vi "Header Fill Check.vi"(8 "error in (no error)":errorcluster, 11 "Sample Properties:":T1) -> (0 "error out":errorcluster, 3 "Cluster":T1)   [LabVIEW 2012]
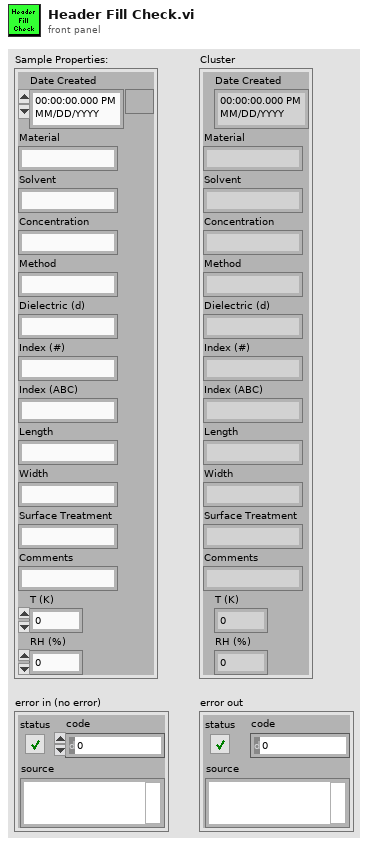
[diagram p1: front panel]
types:
  T1 = cluster{"Date Created":timestamp, "Material":string, "Solvent":string, "Concentration":string, "Method":string, "Dielectric (d)":string, "Index (#)":string, "Index (ABC)":string, "Length":string, "Width":string, "Surface Treatment":string, "Comments":string, "T (K)":dbl, "RH (%)":dbl}
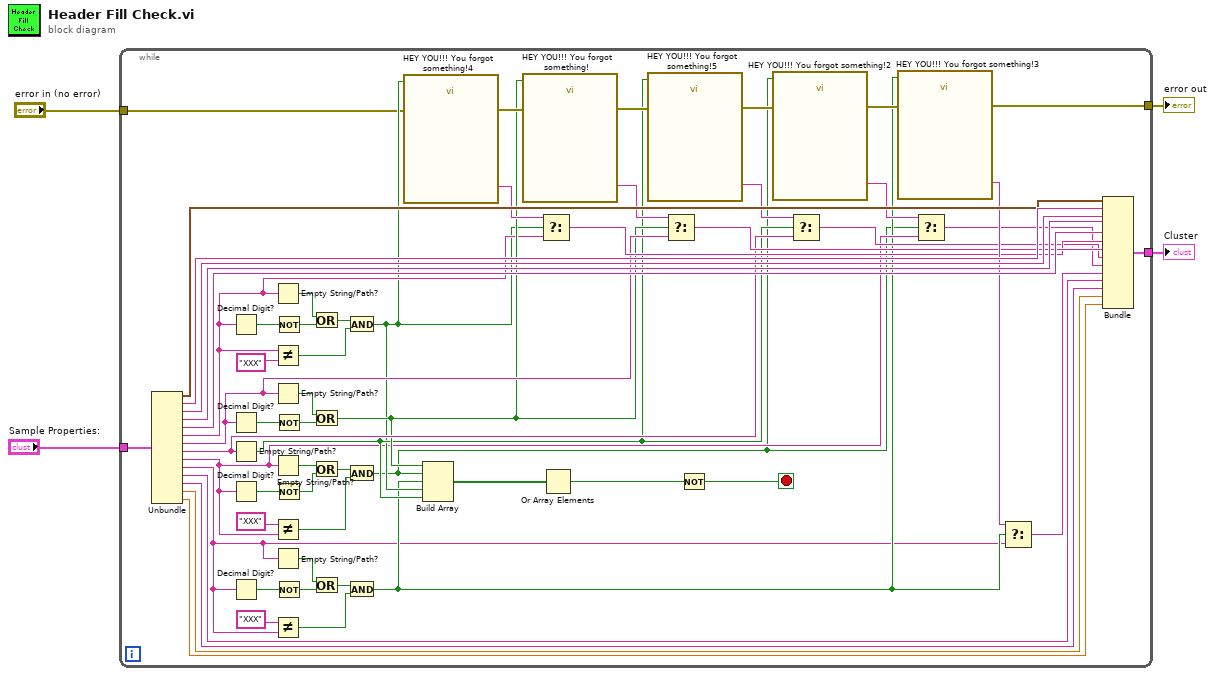
[diagram p0: block diagram]
diagram:
  n1 = while {
    tunnel: "Sample Properties:" -> [w8]
    tunnel: [w7] -> w2
    tunnel: [w6] -> w3
    tunnel: "error in (no error)" -> [w5]
    stop <- w35 stop-if-true
    n2 = Unbundle(w8) -> ("Date Created"=w61:timestamp, "Material"=w62:string, "Solvent"=w63:string, "Concentration"=w64:string, "Method"=w65:string, "Dielectric (d)"=w24:string, "Index (#)"=w52:string, "Index (ABC)"=w49:string, "Length"=w19:string, "Width"=w12:string, "Surface Treatment"=w55:string, "Comments"=w47:string, "T (K)"=w10:dbl, "RH (%)"=w9:dbl)
    n3 = Decimal Digit?(1:w24) -> (0:w32:bool)
    n4 = Decimal Digit?(1:w52) -> (0:w44:bool)
    n5 = Empty String/Path?(string/path=w49) -> (empty?=w38:bool)
    n6 = Decimal Digit?(1:w19) -> (0:w34:bool)
    n7 = Decimal Digit?(1:w12) -> (0:w33:bool)
    n8 = Empty String/Path?(string/path=w24) -> (empty?=w26:bool)
    n9 = Not Equal?(x=w24, y="XXX") -> (x != y?=w23:bool)
    n10 = Empty String/Path?(string/path=w52) -> (empty?=w51:bool)
    n11 = Empty String/Path?(string/path=w19) -> (empty?=w28:bool)
    n12 = Not Equal?(x="XXX", y=w19) -> (x != y?=w18:bool)
    n13 = Empty String/Path?(string/path=w12) -> (empty?=w27:bool)
    n14 = Not Equal?(x="XXX", y=w12) -> (x != y?=w16:bool)
    n15 = Not(x=w32) -> (.not. x?=w29:bool)
    n16 = Not(x=w44) -> (.not. x?=w43:bool)
    n17 = Not(x=w34) -> (.not. x?=w31:bool)
    n18 = Not(x=w33) -> (.not. x?=w30:bool)
    n19 = Or(x=w26, y=w29) -> (x .or. y?=w22:bool)
    n20 = Or(x=w51, y=w43) -> (x .or. y?=w39:bool)
    n21 = Or(x=w28, y=w31) -> (x .or. y?=w17:bool)
    n22 = Or(x=w27, y=w30) -> (x .or. y?=w15:bool)
    n23 = And(x=w22, y=w23) -> (x .and. y?=w21:bool)
    n24 = And(x=w17, y=w18) -> (x .and. y?=w11:bool)
    n25 = And(x=w15, y=w16) -> (x .and. y?=w14:bool)
    n26 = call "HEY YOU!!! You forgot something!4"("Enable"=w21, "error in (no error)"=w5) -> ("Dielectric (d)"=w54:string, "error out"=w40:errorcluster)  [unwired: 15 in, 1 out]
    n27 = Build Array(w39, w11, w14, w21, w38) -> (w37:bool[])
    n28 = call "HEY YOU!!! You forgot something!"("Enable"=w39, "error in (no error)"=w40) -> ("Index (#)"=w60:string, "error out"=w42:errorcluster)  [unwired: 15 in, 1 out]
    n29 = Select(t=w54, s=w21, f=w24) -> (s? t:f=w53:string)
    n30 = Or Array Elements(Boolean array=w37) -> (logical OR=w36:bool)
    n31 = call "HEY YOU!!! You forgot something!5"("Enable"=w38, "error in (no error)"=w42) -> ("Index (ABC)"=w50:string, "error out"=w41:errorcluster)  [unwired: 15 in, 1 out]
    n32 = Select(t=w60, s=w39, f=w52) -> (s? t:f=w57:string)
    n33 = Not(x=w36) -> (.not. x?=w35:bool)
    n34 = call "HEY YOU!!! You forgot something!2"("Enable"=w11, "error in (no error)"=w41) -> ("Length"=w59:string, "error out"=w56:errorcluster)  [unwired: 15 in, 1 out]
    n35 = Select(t=w50, s=w38, f=w49) -> (s? t:f=w48:string)
    n36 = call "HEY YOU!!! You forgot something!3"("Enable"=w14, "error in (no error)"=w56) -> ("Width"=w58:string, "error out"=w6:errorcluster)  [unwired: 15 in, 1 out]
    n37 = Select(t=w59, s=w11, f=w19) -> (s? t:f=w46:string)
    n38 = Select(t=w58, s=w14, f=w12) -> (s? t:f=w45:string)
    n39 = Bundle("Date Created"=w61, "Material"=w62, "Solvent"=w63, "Concentration"=w64, "Method"=w65, "Dielectric (d)"=w53, "Index (#)"=w57, "Index (ABC)"=w48, "Length"=w46, "Width"=w45, "Surface Treatment"=w55, "Comments"=w47, "T (K)"=w10, "RH (%)"=w9) -> (w7:T1)  [unwired: 1 in]
  }
  "error out" <- w3
  "Cluster" <- w2
